vi "PV Revision Query.vi"(8 "error in (no error)":errorcluster, 11 "VISA resource name":refnum<visa-resource-name>) -> (0 "error out":errorcluster, 1 "Software Firmware Revision":string, 2 "Instrument Driver Revision":string, 3 "VISA resource name out":refnum<visa-resource-name>, 4 "Hardware Firmware Revision":string)   [LabVIEW 2016, in "Pfeiffer Vacuum.lvlib"]
doc: "Queries the current instrument firmware revision and instrument driver revision.\n\nRefer to the Readme file for detailed driver information including modification history."
uses:
  Pfeiffer Vacuum.lvlib
panel:
  in  "Adress of unit":u16=1 max=999 step=1
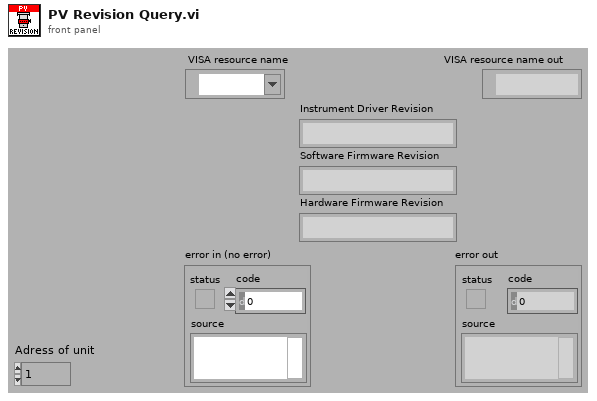
[diagram p1: front panel]
types:
  T1 = cluster{"Major":u16, "Minor":u16, "Fix":u16, "Build":u16}
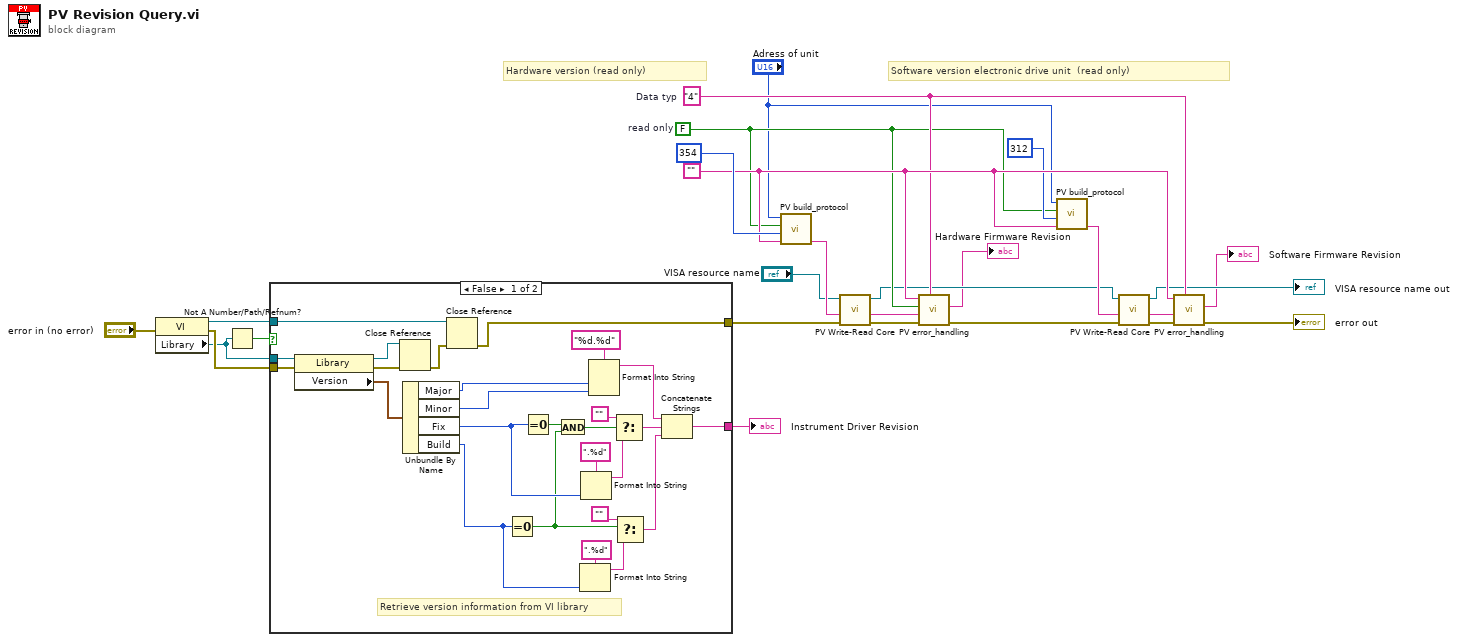
[diagram p0: block diagram]
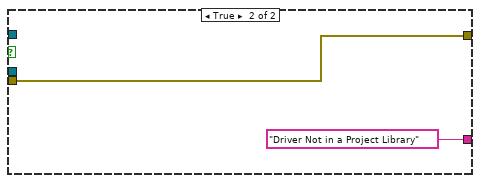
[diagram p2: hidden frame]
diagram:
  w11 = "4"  # Data typ
  w12 = ""
  w9 = FALSE  # read only
  # "Software version electronic drive unit  (read only)"
  # "Hardware version (read only)"
  n1 = property class="VI"(error in="error in (no error)") -> (reference out=w26:refnum<vi>, error out=w25:errorcluster, "Library"=w24:refnum<vi>)  [unwired: 1 in]
  n2 = Not A Number/Path/Refnum?(number/path/refnum=w24) -> (NaN/Path/Refnum?=w23:bool)
  n3 = case shown="False" w23 {
    tunnel: w26 -> [w49 _]
    tunnel: w25 -> [w34 w54]
    tunnel: [w29 w54] -> w16
    tunnel: [w28 "Driver Not in a Project Library"] -> w22
    tunnel: w24 -> [w27 _]
    frame False {
      # "Retrieve version information from VI library"
      n4 = property class="Library"(reference=w27, error in=w34) -> (reference out=w51:refnum<vi>, error out=w52:errorcluster, "Version"=w48:T1)
      n5 = Close Reference(reference=w51, error in (no error)=w52) -> (error out=w50:errorcluster)
      n6 = Unbundle By Name(w48) -> ("Major"=w37:u16, "Minor"=w36:u16, "Fix"=w33:u16, "Build"=w35:u16)
      n7 = Close Reference(reference=w49, error in (no error)=w50) -> (error out=w29:errorcluster)
      n8 = Equal To 0?(x=w35) -> (x = 0?=w31:bool)
      n9 = Equal To 0?(x=w33) -> (x = 0?=w32:bool)
      n10 = And(x=w32, y=w31) -> (x .and. y?=w30:bool)
      n11 = Format Into String(format string=".%d", w35) -> (resulting string=w41:string)  [unwired: 2 in, 1 out]
      n12 = Format Into String(format string=".%d", w33) -> (resulting string=w45:string)  [unwired: 2 in, 1 out]
      n13 = Format Into String(format string="%d.%d", w37, w36) -> (resulting string=w43:string)  [unwired: 2 in, 1 out]
      n14 = Select(t="", s=w30, f=w45) -> (s? t:f=w42:string)
      n15 = Select(t="", s=w31, f=w41) -> (s? t:f=w38:string)
      n16 = Concatenate Strings(w43, w42, w38) -> (w28:string)
    }
    frame True {
    }
  }
  "Instrument Driver Revision" <- w22
  n17 = call "PV build_protocol.vi"("Data"=w12, "Parameter-number"=u16 354, "parameter\nread<->describe"=w9, "Adress"="Adress of unit") -> ("output"=w19:string)  [unwired: 3 in]
  n18 = call "PV Write-Read Core.vi"("error in"=w16, "Write data in"=w19, "VISA session"="VISA resource name") -> ("error out"=w17:errorcluster, "response (data) out"=w18:string, "dup VISA session"=w6:refnum<visa-resource-name>)  [unwired: 2 in]
  n19 = call "PV error_handling.vi"("Data Typ in"=w11, "error in"=w17, "response (data) in"=w18, "Parameter\nread only<->describe"=w9, "data in"=w12) -> ("error out"=w4:errorcluster, "Data out"=→"Hardware Firmware Revision":string)  [unwired: 4 in, 1 out]
  n20 = call "PV build_protocol.vi"("Data"=w12, "Parameter-number"=u16 312, "parameter\nread<->describe"=w9, "Adress"="Adress of unit") -> ("output"=w7:string)  [unwired: 3 in]
  n21 = call "PV Write-Read Core.vi"("error in"=w4, "Write data in"=w7, "VISA session"=w6) -> ("error out"=w14:errorcluster, "response (data) out"=w13:string, "dup VISA session"=→"VISA resource name out":refnum<visa-resource-name>)  [unwired: 2 in]
  n22 = call "PV error_handling.vi"("Data Typ in"=w11, "error in"=w14, "response (data) in"=w13, "data in"=w12) -> ("error out"=→"error out":errorcluster, "Data out"=→"Software Firmware Revision":string)  [unwired: 5 in, 1 out]
